vi "UIM Visibility Configuration.vi"() -> ()   [LabVIEW 2020]
doc: "This example shows that UIM can be used to organize different elements on the UI depending on what is needed at the moment. The user only needs to configure the specific amplitude and frequency so only the appropriate controls are made visible. This way the UI does not need to use tabs to organize elements."
uses:
  UIM Class/UIM.lvclass
  <vilib>/measure/NI_MABase.lvlib
panel:
  in  "Stop Button":bool
  in  "Square Frequency":dbl(knob)=0.9938435865467082 scale=0.0..10.0
  in  "Square Amplitude":dbl(slide)=5.022026431718062 scale=0.0..10.0
  in  "Triangle Frequency":dbl(knob)=1.9305752303119406 scale=0.0..10.0
  in  "Triangle Amplitude":dbl(slide)=6.343612334801763 scale=0.0..10.0
  in  "Sine Frequency":dbl(knob)=5.091919995429821 scale=0.0..10.0
  in  "Sine Amplitude":dbl(slide)=3.876651982378855 scale=0.0..10.0
  out "Waveform Graph":waveform(dbl)[](graph)=[{"t0"=timestamp(131.0 s since 1904-01-01), "dt"=0.001, "Y"=array[1000 elements]}, {"t0"=timestamp(131.0 s since 1904-01-01), "dt"=0.001, "Y"=array[1000 elements]}, {"t0"=timestamp(131.0 s since 1904-01-01), "dt"=0.001, "Y"=array[1000 elements]}]
  in  "Configuration":i32(listbox)
  # "Notice that these settings controls change"
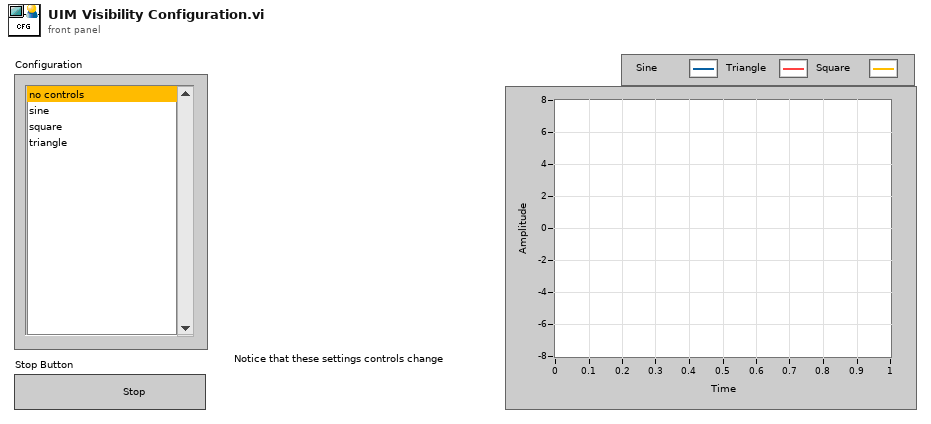
[diagram p1: front panel]
types:
  T1 = enum16{"Sine Wave", "Triangle Wave", "Square Wave", "Sawtooth Wave"}
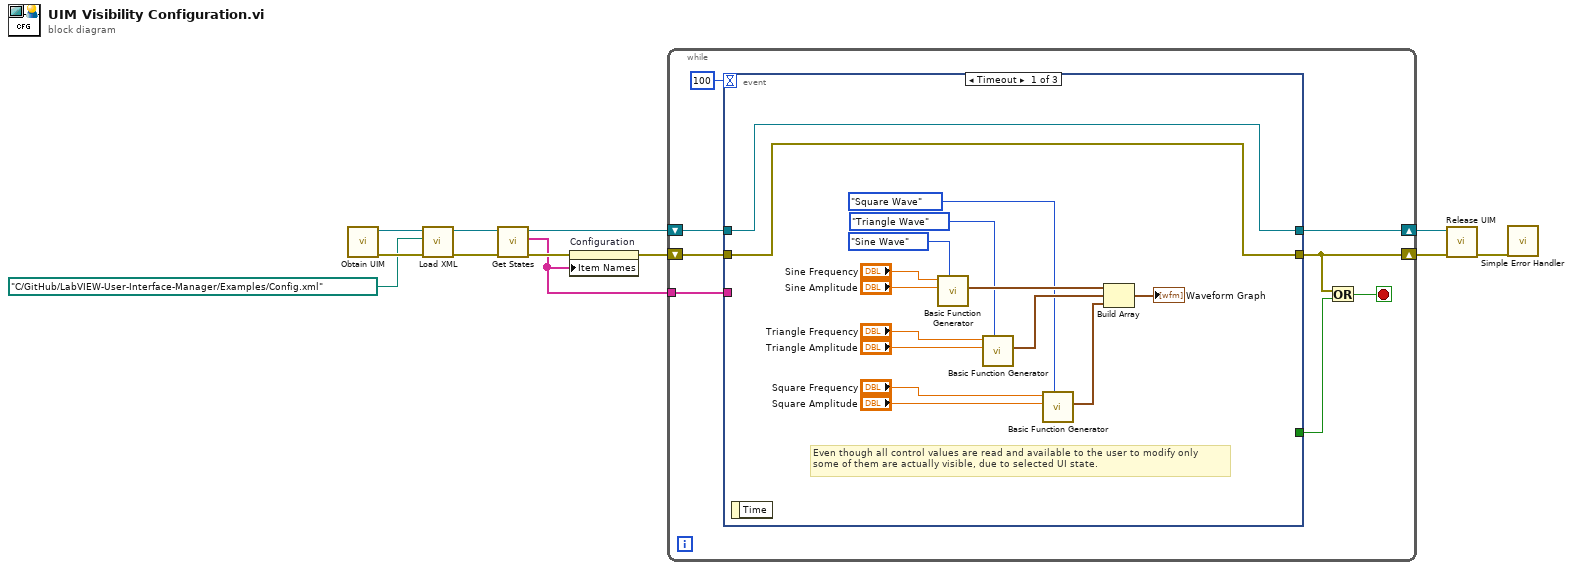
[diagram p0: block diagram]
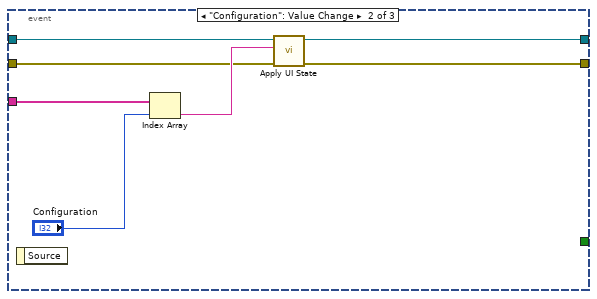
[diagram p2: hidden frame]
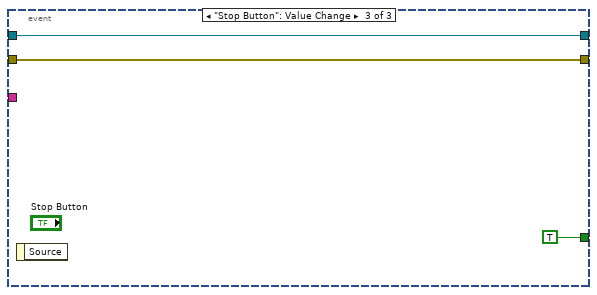
[diagram p3: hidden frame]
diagram:
  n1 = call "Obtain UIM.vi"() -> ("Error Out"=w9:errorcluster, "UIM Handle"=w12:refnum<data-value>)  [unwired: 10 in]
  n2 = call "Load XML.vi"("Error In"=w9, "XML File"=path "C:/GitHub/LabVIEW-User-Interface-Manager/Examples/Config.xml", "UIM In"=w12) -> ("Error Out"=w8:errorcluster, "UIM Out"=w11:refnum<data-value>)  [unwired: 7 in]
  n3 = call "Get States.vi"("Error In"=w8, "UIM In"=w11) -> ("Error Out"=w7:errorcluster, "States"=w5:string[], "UIM Out"=w10:refnum<data-value>)  [unwired: 7 in]
  n4 = property on="Configuration" class="LstBox (strict)"(error in=w7, "Item Names"=w5) -> (error out=w6:errorcluster)  [unwired: 1 in, 1 out]
  n5 = while {
    shift-right: [w13] -> w3
    shift-left: w6 -> [w18]
    shift-right: [w17] -> w4
    shift-left: w10 -> [w19]
    tunnel: w5 -> [w16]
    stop <- w14 stop-if-true
    n6 = event shown="[0] Timeout" {
      selector: _ -> [_ _ _]
      dyn-events: _ -> [_ _ _]
      timeout: 100 -> [_ _ _]
      tunnel: w19 -> [w21 w42 w45]
      tunnel: w18 -> [w22 w37 w44]
      tunnel: [w21 w41 w45] -> w17
      tunnel: w16 -> [_ w40 _]
      tunnel: [w22 w36 w44] -> w13
      tunnel: [_ _ TRUE] -> w15
      event Timeout {
        # "Even though all control values are read and available to the user to modify only\nsome of them are actually visible, due to selected UI state."
        n7 = event-data() -> ()  [unwired: 1 in, 1 out]
        n8 = call <vilib>:"Basic Function Generator.vi"("signal type"=T1."Sine Wave", "amplitude"="Sine Amplitude", "frequency"="Sine Frequency") -> ("signal out"=w26:waveform(dbl))  [unwired: 6 in, 2 out]
        n9 = call <vilib>:"Basic Function Generator.vi"("signal type"=T1."Triangle Wave", "amplitude"="Triangle Amplitude", "frequency"="Triangle Frequency") -> ("signal out"=w27:waveform(dbl))  [unwired: 6 in, 2 out]
        n10 = call <vilib>:"Basic Function Generator.vi"("signal type"=T1."Square Wave", "amplitude"="Square Amplitude", "frequency"="Square Frequency") -> ("signal out"=w28:waveform(dbl))  [unwired: 6 in, 2 out]
        n11 = Build Array(w26, w27, w28) -> (→"Waveform Graph":waveform(dbl)[])
      }
      event "Configuration": Value Change {
        n12 = event-data() -> ()  [unwired: 1 in, 1 out]
        n13 = Index Array(array=w40, index="Configuration") -> (element=w38:string)
        n14 = call "Apply UI State.vi"("Error In"=w37, "State Name"=w38, "UIM In"=w42) -> ("Error Out"=w36:errorcluster, "UIM Out"=w41:refnum<data-value>)  [unwired: 7 in]
      }
      event "Stop Button": Value Change {
        n15 = event-data() -> ()  [unwired: 1 in, 1 out]
      }
    }
    n16 = Or(x=w13, y=w15) -> (x .or. y?=w14:bool)
  }
  n17 = call "Release UIM.vi"("Error In"=w3, "UIM Handle"=w4) -> ("Error Out"=w2:errorcluster)  [unwired: 9 in]
  n18 = call <vilib>:"Simple Error Handler.vi"("error in (no error)"=w2) -> ()  [unwired: 4 in, 5 out]
